vi "spectrogram.vi"() -> ()   [LabVIEW 2012]
doc: "This example demonstrates how to use the STFT Spectrograms VI to analyze the Time-Frequency spectrogram.\n\nInstructions:\n1) Run the VI.\n\n2) Change the <b>time-freq sampling info</b> to see the effect of the different <b>time steps</b> or <b>frequency bins</b> on the spectrogram.\n\n3) Change the window <b>type</b> or <b>length</b> to see the effect of different windows on the spectrogram."
uses:
  Trace controls.ctl
  probe_point.ctl
  pose_selector.ctl
  pose_source.ctl
  pose_relative_to.ctl
  <vilib>/Platform/TimedLoop/XDataNode/timing_clust.ctl
  <vilib>/Platform/TimedLoop/XDataNode/nitl_modes.ctl
  <vilib>/Platform/TimedLoop/XDataNode/wakeup.ctl
  <vilib>/Platform/TimedLoop/XDataNode/XDataNode.xnode
  <vilib>/gmath/NI_Gmath.lvlib
  <vilib>/Platform/TimedLoop/XDataNode/XDNodeRunTimeDep.lvlib
panel:
  out "Cursor time":timestamp
  in  "f max":dbl=200.0 min=100.0 step=100.0
  in  "Pose selectors":T1[](array[typedef])
  in  "dB On":bool=TRUE
  in  "f scaling":bool=TRUE
  in  "stop":bool
  in  "Map selector":T4(ring)=enum."rainbow"
  in  "Selectors":T5[](array[typedef])=[{"+ stim"=FALSE, "Relative"=FALSE, "Scale"=enum."1X", "Probe point"=enum."Position (tip)", "XYZ selector"={"Boolean"=FALSE, "Boolean 2"=FALSE, "Boolean 3"=FALSE}, "To tip"=FALSE}, {"+ stim"=FALSE, "Relative"=FALSE, "Scale"=enum."1X", "Probe point"=enum."Position (tip)", "XYZ selector"={"Boolean"=FALSE, "Boolean 2"=FALSE, "Boolean 3"=FALSE}, "To tip"=FALSE}, {"+ stim"=FALSE, "Relative"=FALSE, "Scale"=enum."1X", "Probe point"=enum."Position (tip)", "XYZ selector"={"Boolean"=FALSE, "Boolean 2"=FALSE, "Boolean 3"=FALSE}, "To tip"=FALSE}, {"+ stim"=FALSE, "Relative"=FALSE, "Scale"=enum."1X", "Probe point"=enum."Position (tip)", "XYZ selector"={"Boolean"=FALSE, "Boolean 2"=FALSE, "Boolean 3"=FALSE}, "To tip"=FALSE}]
  in  "window info":cluster{"type":u32, "length":i32}={"type"=1, "length"=64} {"type" items=["Rectangle"=0, "Hanning"=1, "Hamming"=2, "Blackman-Harris"=3, "Exact Blackman"=4, "Blackman"=5, "Flat Top"=6, "4 Term B-Harris "=7, "7 Term B-Harris"=8, "Low Sidelobe"=9, "Blackman Nuttall"=11, "Triangle"=30, "Gaussian"=62]}
  out "STFT Spectrogram":dbl[][](graph)
  in  "time-freq sampling info":cluster{"time steps":i32, "frequency bins":i32}={"time steps"=4, "frequency bins"=128}
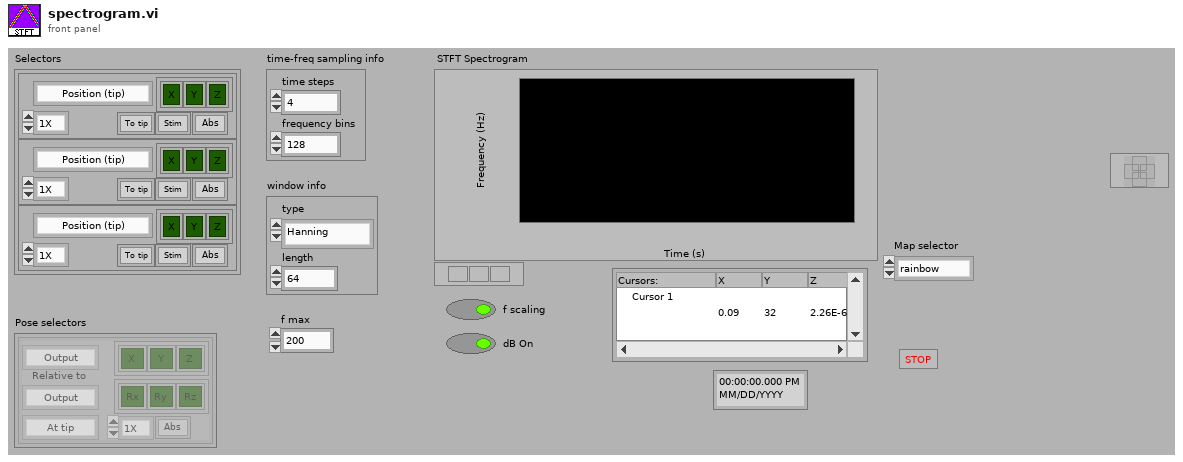
[diagram p1: front panel]
types:
  T1 = typedef "pose_selector.ctl" = cluster{"Scale":enum16{"1X", "10X", "100X", "1KX", "10KX"}, "Source":T2, "XYZ selector":cluster{"Boolean":bool, "Boolean 2":bool, "Boolean 3":bool}, "RPY selector":cluster{"Boolean":bool, "Boolean 2":bool, "Boolean 3":bool}, "Relative to":T3, "Relative":bool, "Translate":enum16{"At tip", "At RCM", "At KC", "At origin"}}
  T2 = typedef "pose_source.ctl" = enum16{"Output", "Handle", "Handle KF", "Goal", "Absolute"}
  T3 = typedef "pose_relative_to.ctl" = enum16{"Output", "Handle", "Handle KF", "Goal", "Absolute", "Trace start"}
  T4 = enum16{"fire", "rainbow", "grey", "inverse grey", "ice", "original"}
  T5 = typedef "Trace controls.ctl" = cluster{"+ stim":bool, "Relative":bool, "Scale":enum16{"1X", "10X", "100X", "1KX", "10KX"}, "Probe point":T6, "XYZ selector":cluster{"Boolean":bool, "Boolean 2":bool, "Boolean 3":bool}, "To tip":bool}
  T6 = typedef "probe_point.ctl" = enum16{"Position (tip)", "Position (RCM)", "Null pos (tip)", "Null pos (RCM)", "V limiter (tip)", "V Limiter (RCM)", "Goal (tip)", "Goal (RCM)", "Link pos 0", "Link pos 1", "KF link pos 0", "KF link pos 1", "Link rate 0", "Link rate 1", "Link residue 0", "Link residue 1", "Link goal 0", "Link goal 1", "Rate limit 0", "Rate limit 1", "Link error 0", "Link error 1", "Controller 0", "Controller 1", "Output 0", "Output 1", "Drive 0", "Drive 1", "Stimulus 0", "Stimulus 1", "Trace data 0", "Trace data 1", "Analog data 0", "Analog data 1", "Status flags", "Light 0", "Light 1", "Light 2", "Light 3", "Light 4", "Light 5", "Goal origin", "Goal rotation 0", "Goal rotation 1", "Goal rotation 2", "Output origin", "Output rotation 0", "Output rotation 1", "Output rotation 2", "Handle origin", "Handle rotation 0", "Handle rotation 1", "Handle rotation 2", "Handle position", "Handle velocity", "Handle acceleration", "Handle angles", "Handle angle rates", "Handle pos residue", "Handle angle residue", "Trace length"}
  T7 = typedef "XDNodeRunTimeDep.lvlib/timing_clust.ctl" = cluster{"Expected End [f-1]":u64, "Actual End [f-1]":u64, "Finished Late? [f-1]":bool, "Expected End [i-1]":u64, "Actual End [i-1]":u64, "Finished Late? [i-1]":bool, "Expected Start [i]":u64, "Actual Start [i]":u64, "Expected Start [f]":u64, "Actual Start [f]":u64, "Source Name":string, "Structure Name":string, "Period":i64, "Deadline":i64, "Offset":i64, "Start":i64, "Priority":i32, "Timeout":i32, "Mode":T8, "Wakeup Reason":T9, "Error":errorcluster, "Source Type":string, "Secondary Source Type":string, "Global End Time":u64, "Global Start Time":u64, "Frame Duration":u64, "Iteration Duration":u64, "Assigned CPU":i32, "I/O Scan Engine Mode":u32}
  T8 = typedef "XDNodeRunTimeDep.lvlib/nitl_modes.ctl" = enum32{"No Change", "Process missed periods, maintain original phase", "Discard missed periods, maintain original phase", "Process missed periods, ignore original phase", "Discard missed periods, ignore original phase"}
  T9 = typedef "XDNodeRunTimeDep.lvlib/wakeup.ctl" = enum32{"Normal", "Aborted", "Asynchronous wakeup", "Timing source error", "Timed loop error", "Timeout"}
  T10 = cluster{"time-freq sampling info":cluster{"time steps":i32, "frequency bins":i32}, "window info":cluster{"type":u32, "length":i32}, "Map selector":enum16{"fire", "rainbow", "grey", "inverse grey", "ice", "original"}, "f scaling":bool, "dB On":bool}
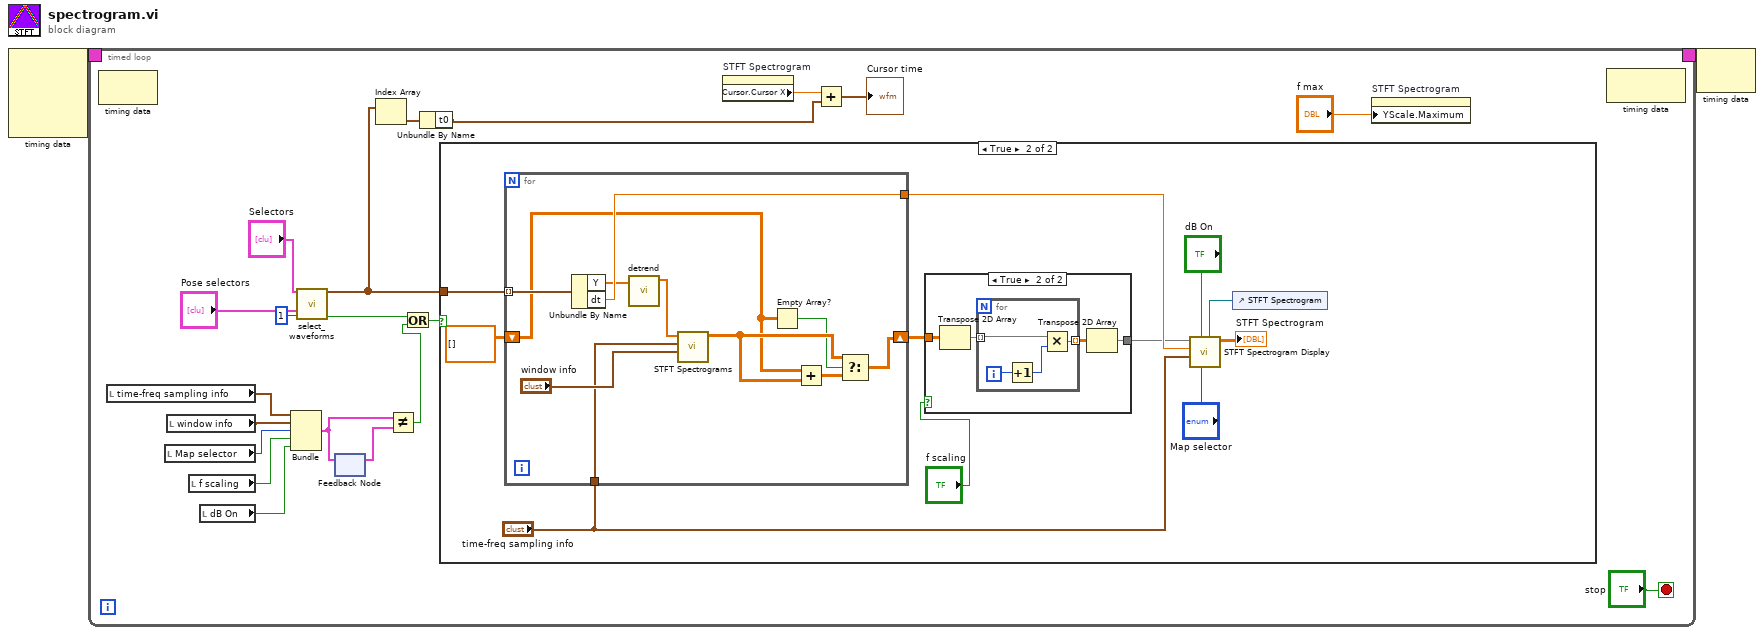
[diagram p0: block diagram]
diagram:
  n1 = node-c288() -> (w2:T7)  [unwired: 4 in]
  n2 = timed-loop {
    timing: w2 -> [_]
    timing-out: [_] -> w1
    stop <- "stop" stop-if-true
    n3 = node-c288() -> ()  [unwired: 1 in, 1 out]
    n4 = local read "time-freq sampling info"() -> (w20:cluster{"time steps":i32, "frequency bins":i32})
    n5 = local read "Map selector"() -> (w13:T4)
    n6 = local read "window info"() -> (w19:cluster{"type":u32, "length":i32})
    n7 = local read "f scaling"() -> (w11:bool)
    n8 = local read "dB On"() -> (w10:bool)
    n9 = Bundle("time-freq sampling info"=w20, "window info"=w19, "Map selector"=w13, "f scaling"=w11, "dB On"=w10) -> (w17:T10)  [unwired: 1 in]
    n10 = call "select_waveforms.vi"("Trace controls"="Selectors", "Pose selectors"="Pose selectors", "Decimate"=1) -> ("Waveforms out"=w7:waveform(sgl)[], "New data"=w16:bool)  [unwired: 9 in, 2 out]
    n11 = feedback-in #1(w17) -> ()
    n12 = feedback #1() -> (w18:T10)  [unwired: 1 in]
    n13 = Index Array(array=w7) -> (element=w6:waveform(sgl))  [unwired: 1 in]
    n14 = Not Equal?(x=w17, y=w18) -> (x != y?=w15:bool)
    n15 = Or(x=w16, y=w15) -> (x .or. y?=w14:bool)
    n16 = Unbundle By Name(w6) -> ("t0"=w4:timestamp)
    n17 = case shown="True" w14 {
      tunnel: w7 -> [_ w33]
      frame False {
      }
      frame True {
        n18 = for {
          tunnel: w33 -> [w52] mode=indexing
          shift-right: [w45] -> w25
          shift-left: dbl[][] [] ("STFT Spectrogram {X}") -> [w47]
          tunnel: [w51] -> w29
          tunnel: "time-freq sampling info" -> [w50]
          n19 = Unbundle By Name(w52) -> ("Y"=w44:sgl[], "dt"=w51:dbl)
          n20 = call "detrend.vi"("Array in"=w44) -> ("Array out"=w43:sgl[])  [unwired: 10 in]
          n21 = call <vilib>:"STFT Spectrograms.vi"("window info"="window info", "time-freq sampling info"=w50, "X"=w43) -> ("STFT Spectrogram {X}"=w48:dbl[][])  [unwired: 3 in, 5 out]
          n22 = Empty Array?(array=w47) -> (empty?=w46:bool)
          n23 = Add(x=w47, y=w48) -> (x+y=w49:dbl[][])
          n24 = Select(t=w48, s=w46, f=w49) -> (s? t:f=w45:dbl[][])
        }
        n25 = case shown="True" "f scaling" {
          tunnel: w25 -> [w34 w38]
          tunnel: [w34 w35] -> w24
          frame False {
          }
          frame True {
            n26 = Transpose 2D Array(2D array=w38) -> (transposed array=w37:dbl[][])
            n27 = for {
              tunnel: w37 -> [w40] mode=indexing
              tunnel: [w39] -> w36 mode=indexing
              i -> [w42]
              n28 = Increment(x=w42) -> (x+1=w41:i32)
              n29 = Multiply(x=w40, y=w41) -> (x*y=w39:dbl[])
            }
            n30 = Transpose 2D Array(2D array=w36) -> (transposed array=w35:dbl[][])
          }
        }
        n31 = control-ref of="STFT Spectrogram"() -> (w30:refnum<vi>)
        n32 = call "STFT Spectrogram Display.vi"("Intensity Graph"=w30, "map selector"="Map selector", "dB On"="dB On", "time-freq sampling info"="time-freq sampling info", "dt"=w29, "STFT Spectrogram In"=w24) -> ("STFT Spectrogram Out"=→"STFT Spectrogram":dbl[][])  [unwired: 1 in, 4 out]
      }
    }
    n33 = property on="STFT Spectrogram" class="IntGraph (strict)"() -> ("Cursor.Cursor X"=w3:dbl)  [unwired: 2 in, 2 out]
    n34 = Add(x=w3, y=w4) -> (x+y=→"Cursor time":timestamp)
    n35 = property on="STFT Spectrogram" class="IntGraph (strict)"("YScale.Maximum"="f max") -> ()  [unwired: 2 in, 2 out]
    n36 = node-c288() -> ()  [unwired: 1 in, 1 out]
  }
  n37 = node-c288(w1) -> ()  [unwired: 1 out]
